vi "CloseConfigFile.vi"(8 "error in (no error)":errorcluster, 11 "refnum":T1) -> (0 "error out":errorcluster, 3 "file path":path)   [LabVIEW 2020, in "ViewableActor.lvlib"]
doc: "Writes data to the platform-independent configuration file identified by <B>refnum</B> and then closes the reference to that file."
uses:
  ViewableActor.lvlib
  <vilib>/Utility/config.llb/Config Data RefNum.ctl
  <vilib>/Utility/config.llb/NI_LVConfig.lvlib
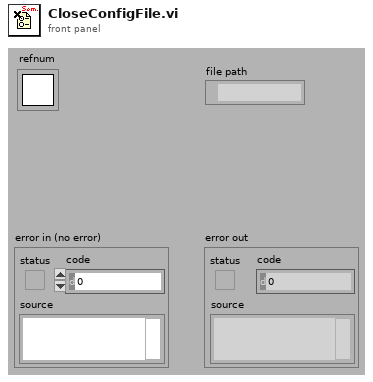
[diagram p1: front panel]
types:
  T1 = typedef "NI_LVConfig.lvlib/Config Data RefNum.ctl" = refnum<k1>
  T2 = typedef "Semaphore RefNum" = refnum<k1>
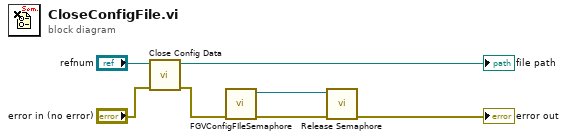
[diagram p0: block diagram]
diagram:
  n1 = call <vilib>:"Close Config Data.vi"("error in (no error)"="error in (no error)", "refnum"="refnum") -> ("error out"=w5:errorcluster, "file path"=→"file path":path)  [unwired: 8 in]
  n2 = call "FGVConfigFIleSemaphore.vi"("error in (no error)"=w5) -> ("error out"=w3:errorcluster, "semaphore"=w4:T2)  [unwired: 9 in]
  n3 = call <vilib>:"Release Semaphore.vi"("error in (no error)"=w3, "semaphore"=w4) -> ("error out"=→"error out":errorcluster)  [unwired: 4 in, 1 out]
